vi "Write To .dat File.vi"(10 "Frame Number":u32, 11 ".dat File":refnum<file>) -> (3 ".dat File (Duplicate)":refnum<file>)   [LabVIEW 2014]
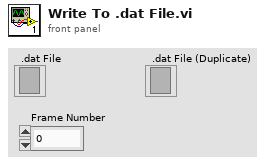
[diagram p1: front panel]
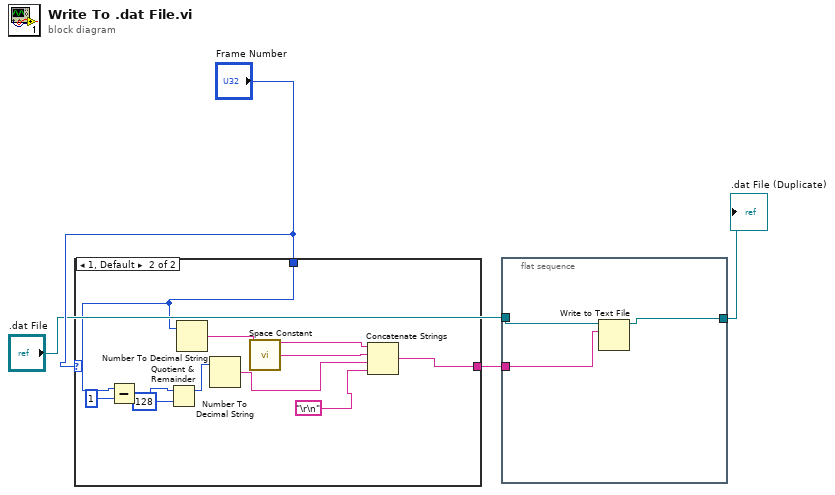
[diagram p0: block diagram]
diagram:
  n1 = case shown="1, Default" "Frame Number" {
    tunnel: [_ w12] -> w2
    tunnel: "Frame Number" -> [_ w11]
    frame 0 {
    }
    frame 1, Default {
      n2 = Subtract(x=w11, y=u32 1) -> (x-y=w9:u32)
      n3 = Quotient & Remainder(x=w9, y=u32 128) -> (x-y*floor(x/y)=w7:u32)  [unwired: 1 out]
      n4 = Number To Decimal String(number=w11) -> (decimal integer string=w13:string)  [unwired: 1 in]
      n5 = Number To Decimal String(number=w7) -> (decimal integer string=w6:string)  [unwired: 1 in]
      n6 = call <vilib>:"Space Constant.vi"() -> ("String"=w14:string)
      n7 = Concatenate Strings "Concatenate Strings"(w13, w14, w6, "\r\n") -> (w12:string)
    }
  }
  n8 = flat-sequence {
    tunnel: ".dat File" -> [w17]
    tunnel: w2 -> [w16]
    tunnel: [w15] -> w3
    frame #0 {
      n9 = Write to Text File(file (use dialog)=w17, text=w16) -> (refnum out=w15:refnum<file>)  [unwired: 2 in, 2 out]
    }
  }
  ".dat File (Duplicate)" <- w3
